vi "Nested Status.vi"(11 "Ex Queue Actor in":refnum<class "Ex Queue Actor.lvclass">) -> (0 "Nested Count":i32, 1 "Nested Aliases":string[](array[string]), 2 "Any Exist?":bool)   [LabVIEW 2021, in "Ex Queue Actor.lvlib" / "Ex Queue Actor.lvclass"]
uses:
  Ex Queue Actor.lvclass
  Ex Queue Actor.lvclass/Ex Queue Actor.ctl
  Actor/Queue Actor/Queue Actor.lvclass
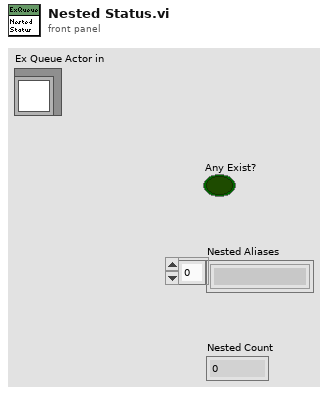
[diagram p1: front panel]
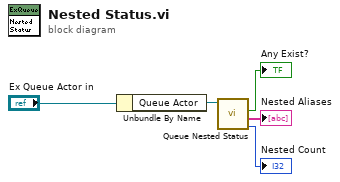
[diagram p0: block diagram]
diagram:
  n1 = Unbundle By Name("Ex Queue Actor in") -> ("Queue Actor"=w4:refnum<class "Queue Actor.lvclass">)
  n2 = call-dynamic "Queue Nested Status.vi"("Actor in"=w4) -> ("Queue Nested Count"=→"Nested Count":i32, "Queue Nested Aliases"=→"Nested Aliases":string[], "Any Exist?"=→"Any Exist?":bool)  [unwired: 8 in]
